vi "Register gRPC Messages.vi"(8 "error in (no error)":errorcluster, 11 "gRPC ID":T1) -> (0 "error out":errorcluster, 3 "gRPC ID Out":T1)   [LabVIEW 2025, in "xnet_can_bus_monitor_api_server.lvlib"]
uses:
  xnet_can_bus_monitor_api_server.lvlib
  <vilib>/gRPC/LabVIEW gRPC Library/Shared/grpcId.ctl
  <vilib>/gRPC/LabVIEW gRPC Library/Server API/typeDefs/Message Metadata.ctl
  <vilib>/gRPC/LabVIEW gRPC Library/Server API/typeDefs/Message Element Metadata.ctl
  <vilib>/gRPC/LabVIEW gRPC Library/Server API/typeDefs/Message Element Type.ctl
  <vilib>/gRPC/LabVIEW gRPC Library/Server API/typeDefs/Enum Metadata.ctl
  <vilib>/gRPC/LabVIEW gRPC Library/grpc-lvsupport-release.lvlib
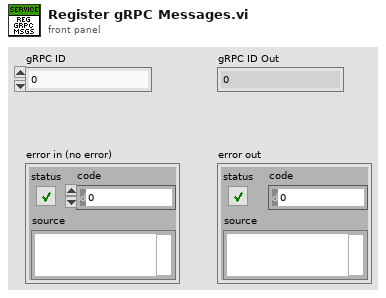
[diagram p1: front panel]
types:
  T1 = typedef "grpc-lvsupport-release.lvlib/grpcId.ctl" = u64
  T2 = typedef "grpc-lvsupport-release.lvlib/Enum Metadata.ctl" = cluster{"Version":i32, "Name":string, "Type Url":string, "Enum Values":string, "Allow Alias":bool}
  T3 = typedef "grpc-lvsupport-release.lvlib/Message Metadata.ctl" = cluster{"Version":i32, "Name":string, "Type Url":string, "Elements":T4[], "Has Oneof":bool}
  T4 = typedef "grpc-lvsupport-release.lvlib/Message Element Metadata.ctl" = cluster{"Field Name":string, "Embedded Message Name":string, "Protobuf Index":i32, "MessageElementType":T5, "Repeated":bool, "Is in Oneof":bool, "Oneof Container Name":string}
  T5 = typedef "grpc-lvsupport-release.lvlib/Message Element Type.ctl" = enum32{"Int32Value", "FloatValue", "DoubleValue", "BoolValue", "StringValue", "MessageValue", "Int64Value", "UInt32Value", "UInt64Value", "EnumValue", "Bytes", "Fixed64", "Fixed32", "SFixed64", "SFixed32", "SInt64", "SInt32"}
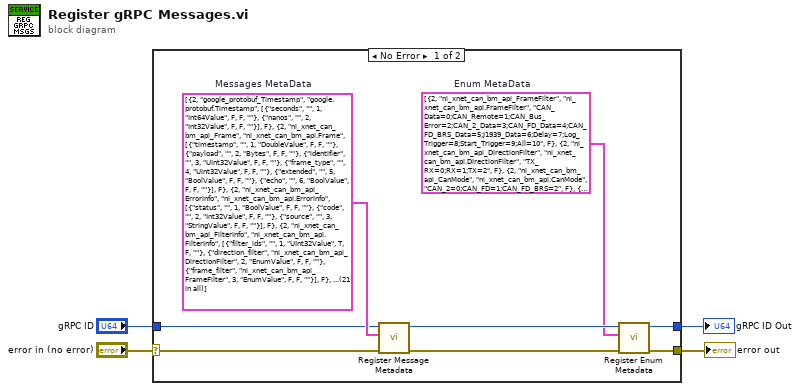
[diagram p0: block diagram]
diagram:
  n1 = case shown="No Error" "error in (no error)" {
    selector: "error in (no error)" -> [w10 w13]
    tunnel: [w9 w12] -> w2
    tunnel: [w6 w13] -> w1
    tunnel: "gRPC ID" -> [w9 w12]
    frame No Error {
      w5 = T2[] [{"Version"=2, "Name"="ni_xnet_can_bm_api_FrameFilter", "Type Url"="ni_xnet_can_bm_api.FrameFilter", "Enum Values"="CAN_Data=0;CAN_Remote=1;CAN_Bus_Error=2;CAN_2_Data=3;CAN_FD_Data=4;CAN_FD_BRS_Data=5;J1939_Data=6;Delay=7;Log_Trigger=8;Start_Trigger=9;All=10", "Allow Alias"=FALSE}, {"Version"=2, "Name"="ni_xnet_can_bm_api_DirectionFilter", "Type Url"="ni_xnet_can_bm_api.DirectionFilter", "Enum Values"="TX_RX=0;RX=1;TX=2", "Allow Alias"=FALSE}, {"Version"=2, "Name"="ni_xnet_can_bm_api_CanMode", "Type Url"="ni_xnet_can_bm_api.CanMode", "Enum Values"="CAN_2=0;CAN_FD=1;CAN_FD_BRS=2", "Allow Alias"=FALSE}, {"Version"=2, "Name"="ni_xnet_can_bm_api_CommState", "Type Url"="ni_xnet_can_bm_api.CommState", "Enum Values"="Error_Active=0;Error_Passive=1;Bus_Off=2;Init=3", "Allow Alias"=FALSE}, {"Version"=2, "Name"="ni_xnet_can_bm_api_LastCommError", "Type Url"="ni_xnet_can_bm_api.LastCommError", "Enum Values"="None=0;Stuff=1;Form=2;ACK=3;Bit1=4;Bit0=5;CRC=6", "Allow Alias"=FALSE}, {"Version"=2, "Name"="ni_xnet_can_bm_api_FdIsoMode", "Type Url"="ni_xnet_can_bm_api.FdIsoMode", "Enum Values"="ISO=0;Non_ISO=1;ISO_Legacy=2", "Allow Alias"=FALSE}, {"Version"=2, "Name"="ni_xnet_can_bm_api_Termination", "Type Url"="ni_xnet_can_bm_api.Termination", "Enum Values"="Term_Off=0;Term_On=1", "Allow Alias"=FALSE}]  # Enum MetaData
      w11 = T3[] [{"Version"=2, "Name"="google_protobuf_Timestamp", "Type Url"="google.protobuf.Timestamp", "Elements"=[{"Field Name"="seconds", "Embedded Message Name"="", "Protobuf Index"=1, "MessageElementType"=enum."Int64Value", "Repeated"=FALSE, "Is in Oneof"=FALSE, "Oneof Container Name"=""}, {"Field Name"="nanos", "Embedded Message Name"="", "Protobuf Index"=2, "MessageElementType"=enum."Int32Value", "Repeated"=FALSE, "Is in Oneof"=FALSE, "Oneof Container Name"=""}], "Has Oneof"=FALSE}, {"Version"=2, "Name"="ni_xnet_can_bm_api_Frame", "Type Url"="ni_xnet_can_bm_api.Frame", "Elements"=[{"Field Name"="timestamp", "Embedded Message Name"="", "Protobuf Index"=1, "MessageElementType"=enum."DoubleValue", "Repeated"=FALSE, "Is in Oneof"=FALSE, "Oneof Container Name"=""}, {"Field Name"="payload", "Embedded Message Name"="", "Protobuf Index"=2, "MessageElementType"=enum."Bytes", "Repeated"=FALSE, "Is in Oneof"=FALSE, "Oneof Container Name"=""}, {"Field Name"="identifier", "Embedded Message Name"="", "Protobuf Index"=3, "MessageElementType"=enum."UInt32Value", "Repeated"=FALSE, "Is in Oneof"=FALSE, "Oneof Container Name"=""}, {"Field Name"="frame_type", "Embedded Message Name"="", "Protobuf Index"=4, "MessageElementType"=enum."UInt32Value", "Repeated"=FALSE, "Is in Oneof"=FALSE, "Oneof Container Name"=""}, {"Field Name"="extended", "Embedded Message Name"="", "Protobuf Index"=5, "MessageElementType"=enum."BoolValue", "Repeated"=FALSE, "Is in Oneof"=FALSE, "Oneof Container Name"=""}, {"Field Name"="echo", "Embedded Message Name"="", "Protobuf Index"=6, "MessageElementType"=enum."BoolValue", "Repeated"=FALSE, "Is in Oneof"=FALSE, "Oneof Container Name"=""}], "Has Oneof"=FALSE}, {"Version"=2, "Name"="ni_xnet_can_bm_api_ErrorInfo", "Type Url"="ni_xnet_can_bm_api.ErrorInfo", "Elements"=[{"Field Name"="status", "Embedded Message Name"="", "Protobuf Index"=1, "MessageElementType"=enum."BoolValue", "Repeated"=FALSE, "Is in Oneof"=FALSE, "Oneof Container Name"=""}, {"Field Name"="code", "Embedded Message Name"="", "Protobuf Index"=2, "MessageElementType"=enum."Int32Value", "Repeated"=FALSE, "Is in Oneof"=FALSE, "Oneof Container Name"=""}, {"Field Name"="source", "Embedded Message Name"="", "Protobuf Index"=3, "MessageElementType"=enum."StringValue", "Repeated"=FALSE, "Is in Oneof"=FALSE, "Oneof Container Name"=""}], "Has Oneof"=FALSE}, {"Version"=2, "Name"="ni_xnet_can_bm_api_FilterInfo", "Type Url"="ni_xnet_can_bm_api.FilterInfo", "Elements"=[{"Field Name"="filter_ids", "Embedded Message Name"="", "Protobuf Index"=1, "MessageElementType"=enum."UInt32Value", "Repeated"=TRUE, "Is in Oneof"=FALSE, "Oneof Container Name"=""}, {"Field Name"="direction_filter", "Embedded Message Name"="ni_xnet_can_bm_api_DirectionFilter", "Protobuf Index"=2, "MessageElementType"=enum."EnumValue", "Repeated"=FALSE, "Is in Oneof"=FALSE, "Oneof Container Name"=""}, {"Field Name"="frame_filter", "Embedded Message Name"="ni_xnet_can_bm_api_FrameFilter", "Protobuf Index"=3, "MessageElementType"=enum."EnumValue", "Repeated"=FALSE, "Is in Oneof"=FALSE, "Oneof Container Name"=""}], "Has Oneof"=FALSE}, {"Version"=2, "Name"="ni_xnet_can_bm_api_ConnectSettings", "Type Url"="ni_xnet_can_bm_api.ConnectSettings", "Elements"=[{"Field Name"="port", "Embedded Message Name"="", "Protobuf Index"=1, "MessageElementType"=enum."StringValue", "Repeated"=FALSE, "Is in Oneof"=FALSE, "Oneof Container Name"=""}, {"Field Name"="can_mode", "Embedded Message Name"="ni_xnet_can_bm_api_CanMode", "Protobuf Index"=2, "MessageElementType"=enum."EnumValue", "Repeated"=FALSE, "Is in Oneof"=FALSE, "Oneof Container Name"=""}, {"Field Name"="termination", "Embedded Message Name"="ni_xnet_can_bm_api_Termination", "Protobuf Index"=3, "MessageElementType"=enum."EnumValue", "Repeated"=FALSE, "Is in Oneof"=FALSE, "Oneof Container Name"=""}, {"Field Name"="baud_rate", "Embedded Message Name"="", "Protobuf Index"=4, "MessageElementType"=enum."UInt64Value", "Repeated"=FALSE, "Is in Oneof"=FALSE, "Oneof Container Name"=""}, {"Field Name"="fd_baud_rate", "Embedded Message Name"="", "Protobuf Index"=5, "MessageElementType"=enum."UInt64Value", "Repeated"=FALSE, "Is in Oneof"=FALSE, "Oneof Container Name"=""}, {"Field Name"="fd_iso_mode", "Embedded Message Name"="ni_xnet_can_bm_api_FdIsoMode", "Protobuf Index"=6, "MessageElementType"=enum."EnumValue", "Repeated"=FALSE, "Is in Oneof"=FALSE, "Oneof Container Name"=""}], "Has Oneof"=FALSE}, {"Version"=2, "Name"="ni_xnet_can_bm_api_CanCommState", "Type Url"="ni_xnet_can_bm_api.CanCommState", "Elements"=[{"Field Name"="fault_code", "Embedded Message Name"="", "Protobuf Index"=1, "MessageElementType"=enum."Int32Value", "Repeated"=FALSE, "Is in Oneof"=FALSE, "Oneof Container Name"=""}, {"Field Name"="fault", "Embedded Message Name"="", "Protobuf Index"=2, "MessageElementType"=enum."BoolValue", "Repeated"=FALSE, "Is in Oneof"=FALSE, "Oneof Container Name"=""}, {"Field Name"="comm_state", "Embedded Message Name"="ni_xnet_can_bm_api_CommState", "Protobuf Index"=3, "MessageElementType"=enum."EnumValue", "Repeated"=FALSE, "Is in Oneof"=FALSE, "Oneof Container Name"=""}, {"Field Name"="last_comm_error", "Embedded Message Name"="ni_xnet_can_bm_api_LastCommError", "Protobuf Index"=4, "MessageElementType"=enum."EnumValue", "Repeated"=FALSE, "Is in Oneof"=FALSE, "Oneof Container Name"=""}, {"Field Name"="receive_error_counter", "Embedded Message Name"="", "Protobuf Index"=5, "MessageElementType"=enum."UInt32Value", "Repeated"=FALSE, "Is in Oneof"=FALSE, "Oneof Container Name"=""}, {"Field Name"="transmit_error_counter", "Embedded Message Name"="", "Protobuf Index"=6, "MessageElementType"=enum."UInt32Value", "Repeated"=FALSE, "Is in Oneof"=FALSE, "Oneof Container Name"=""}, {"Field Name"="transceiver_error", "Embedded Message Name"="", "Protobuf Index"=7, "MessageElementType"=enum."BoolValue", "Repeated"=FALSE, "Is in Oneof"=FALSE, "Oneof Container Name"=""}, {"Field Name"="sleep", "Embedded Message Name"="", "Protobuf Index"=8, "MessageElementType"=enum."BoolValue", "Repeated"=FALSE, "Is in Oneof"=FALSE, "Oneof Container Name"=""}], "Has Oneof"=FALSE}, {"Version"=2, "Name"="ni_xnet_can_bm_api_Session", "Type Url"="ni_xnet_can_bm_api.Session", "Elements"=[{"Field Name"="name", "Embedded Message Name"="", "Protobuf Index"=1, "MessageElementType"=enum."StringValue", "Repeated"=FALSE, "Is in Oneof"=FALSE, "Oneof Container Name"=""}, {"Field Name"="session_uid", "Embedded Message Name"="", "Protobuf Index"=2, "MessageElementType"=enum."StringValue", "Repeated"=FALSE, "Is in Oneof"=FALSE, "Oneof Container Name"=""}], "Has Oneof"=FALSE}, {"Version"=2, "Name"="ni_xnet_can_bm_api_PassThruRequest", "Type Url"="ni_xnet_can_bm_api.PassThruRequest", "Elements"=[{"Field Name"="session", "Embedded Message Name"="ni_xnet_can_bm_api_Session", "Protobuf Index"=1, "MessageElementType"=enum."MessageValue", "Repeated"=FALSE, "Is in Oneof"=FALSE, "Oneof Container Name"=""}, {"Field Name"="frame", "Embedded Message Name"="ni_xnet_can_bm_api_Frame", "Protobuf Index"=2, "MessageElementType"=enum."MessageValue", "Repeated"=FALSE, "Is in Oneof"=FALSE, "Oneof Container Name"=""}], "Has Oneof"=FALSE}, {"Version"=2, "Name"="ni_xnet_can_bm_api_PassThruReply", "Type Url"="ni_xnet_can_bm_api.PassThruReply", "Elements"=[{"Field Name"="error", "Embedded Message Name"="ni_xnet_can_bm_api_ErrorInfo", "Protobuf Index"=1, "MessageElementType"=enum."MessageValue", "Repeated"=FALSE, "Is in Oneof"=FALSE, "Oneof Container Name"=""}], "Has Oneof"=FALSE}, {"Version"=2, "Name"="ni_xnet_can_bm_api_GetStreamingFilterRequest", "Type Url"="ni_xnet_can_bm_api.GetStreamingFilterRequest", "Elements"=[{"Field Name"="session", "Embedded Message Name"="ni_xnet_can_bm_api_Session", "Protobuf Index"=1, "MessageElementType"=enum."MessageValue", "Repeated"=FALSE, "Is in Oneof"=FALSE, "Oneof Container Name"=""}], "Has Oneof"=FALSE}, {"Version"=2, "Name"="ni_xnet_can_bm_api_GetStreamingFilterReply", "Type Url"="ni_xnet_can_bm_api.GetStreamingFilterReply", "Elements"=[{"Field Name"="filter_info", "Embedded Message Name"="ni_xnet_can_bm_api_FilterInfo", "Protobuf Index"=1, "MessageElementType"=enum."MessageValue", "Repeated"=FALSE, "Is in Oneof"=FALSE, "Oneof Container Name"=""}, {"Field Name"="error", "Embedded Message Name"="ni_xnet_can_bm_api_ErrorInfo", "Protobuf Index"=2, "MessageElementType"=enum."MessageValue", "Repeated"=FALSE, "Is in Oneof"=FALSE, "Oneof Container Name"=""}], "Has Oneof"=FALSE}, {"Version"=2, "Name"="ni_xnet_can_bm_api_SetStreamingFilterRequest", "Type Url"="ni_xnet_can_bm_api.SetStreamingFilterRequest", "Elements"=[{"Field Name"="session", "Embedded Message Name"="ni_xnet_can_bm_api_Session", "Protobuf Index"=1, "MessageElementType"=enum."MessageValue", "Repeated"=FALSE, "Is in Oneof"=FALSE, "Oneof Container Name"=""}, {"Field Name"="filter_info", "Embedded Message Name"="ni_xnet_can_bm_api_FilterInfo", "Protobuf Index"=2, "MessageElementType"=enum."MessageValue", "Repeated"=FALSE, "Is in Oneof"=FALSE, "Oneof Container Name"=""}], "Has Oneof"=FALSE}, {"Version"=2, "Name"="ni_xnet_can_bm_api_SetStreamingFilterReply", "Type Url"="ni_xnet_can_bm_api.SetStreamingFilterReply", "Elements"=[{"Field Name"="error", "Embedded Message Name"="ni_xnet_can_bm_api_ErrorInfo", "Protobuf Index"=1, "MessageElementType"=enum."MessageValue", "Repeated"=FALSE, "Is in Oneof"=FALSE, "Oneof Container Name"=""}], "Has Oneof"=FALSE}, {"Version"=2, "Name"="ni_xnet_can_bm_api_ResetStreamingFilterRequest", "Type Url"="ni_xnet_can_bm_api.ResetStreamingFilterRequest", "Elements"=[{"Field Name"="session", "Embedded Message Name"="ni_xnet_can_bm_api_Session", "Protobuf Index"=1, "MessageElementType"=enum."MessageValue", "Repeated"=FALSE, "Is in Oneof"=FALSE, "Oneof Container Name"=""}], "Has Oneof"=FALSE}, {"Version"=2, "Name"="ni_xnet_can_bm_api_ResetStreamingFilterReply", "Type Url"="ni_xnet_can_bm_api.ResetStreamingFilterReply", "Elements"=[{"Field Name"="filter_info", "Embedded Message Name"="ni_xnet_can_bm_api_FilterInfo", "Protobuf Index"=1, "MessageElementType"=enum."MessageValue", "Repeated"=FALSE, "Is in Oneof"=FALSE, "Oneof Container Name"=""}, {"Field Name"="error", "Embedded Message Name"="ni_xnet_can_bm_api_ErrorInfo", "Protobuf Index"=2, "MessageElementType"=enum."MessageValue", "Repeated"=FALSE, "Is in Oneof"=FALSE, "Oneof Container Name"=""}], "Has Oneof"=FALSE}, {"Version"=2, "Name"="ni_xnet_can_bm_api_InitializeSettingsRequest", "Type Url"="ni_xnet_can_bm_api.InitializeSettingsRequest", "Elements"=[{"Field Name"="name", "Embedded Message Name"="", "Protobuf Index"=1, "MessageElementType"=enum."StringValue", "Repeated"=FALSE, "Is in Oneof"=FALSE, "Oneof Container Name"=""}, {"Field Name"="connect_settings", "Embedded Message Name"="ni_xnet_can_bm_api_ConnectSettings", "Protobuf Index"=2, "MessageElementType"=enum."MessageValue", "Repeated"=FALSE, "Is in Oneof"=FALSE, "Oneof Container Name"=""}, {"Field Name"="default_filter_ids", "Embedded Message Name"="", "Protobuf Index"=3, "MessageElementType"=enum."UInt32Value", "Repeated"=TRUE, "Is in Oneof"=FALSE, "Oneof Container Name"=""}], "Has Oneof"=FALSE}, {"Version"=2, "Name"="ni_xnet_can_bm_api_InitializeSettingsReply", "Type Url"="ni_xnet_can_bm_api.InitializeSettingsReply", "Elements"=[{"Field Name"="session", "Embedded Message Name"="ni_xnet_can_bm_api_Session", "Protobuf Index"=1, "MessageElementType"=enum."MessageValue", "Repeated"=FALSE, "Is in Oneof"=FALSE, "Oneof Container Name"=""}, {"Field Name"="error", "Embedded Message Name"="ni_xnet_can_bm_api_ErrorInfo", "Protobuf Index"=2, "MessageElementType"=enum."MessageValue", "Repeated"=FALSE, "Is in Oneof"=FALSE, "Oneof Container Name"=""}], "Has Oneof"=FALSE}, {"Version"=2, "Name"="ni_xnet_can_bm_api_StopProcessRequest", "Type Url"="ni_xnet_can_bm_api.StopProcessRequest", "Elements"=[{"Field Name"="session", "Embedded Message Name"="ni_xnet_can_bm_api_Session", "Protobuf Index"=1, "MessageElementType"=enum."MessageValue", "Repeated"=FALSE, "Is in Oneof"=FALSE, "Oneof Container Name"=""}], "Has Oneof"=FALSE}, {"Version"=2, "Name"="ni_xnet_can_bm_api_StopProcessReply", "Type Url"="ni_xnet_can_bm_api.StopProcessReply", "Elements"=[{"Field Name"="stopped", "Embedded Message Name"="", "Protobuf Index"=1, "MessageElementType"=enum."BoolValue", "Repeated"=FALSE, "Is in Oneof"=FALSE, "Oneof Container Name"=""}, {"Field Name"="error", "Embedded Message Name"="ni_xnet_can_bm_api_ErrorInfo", "Protobuf Index"=2, "MessageElementType"=enum."MessageValue", "Repeated"=FALSE, "Is in Oneof"=FALSE, "Oneof Container Name"=""}], "Has Oneof"=FALSE}, {"Version"=2, "Name"="ni_xnet_can_bm_api_StreamBusRequest", "Type Url"="ni_xnet_can_bm_api.StreamBusRequest", "Elements"=[{"Field Name"="session", "Embedded Message Name"="ni_xnet_can_bm_api_Session", "Protobuf Index"=1, "MessageElementType"=enum."MessageValue", "Repeated"=FALSE, "Is in Oneof"=FALSE, "Oneof Container Name"=""}], "Has Oneof"=FALSE}, {"Version"=2, "Name"="ni_xnet_can_bm_api_StreamBusReply", "Type Url"="ni_xnet_can_bm_api.StreamBusReply", "Elements"=[{"Field Name"="can_comm_state", "Embedded Message Name"="ni_xnet_can_bm_api_CanCommState", "Protobuf Index"=1, "MessageElementType"=enum."MessageValue", "Repeated"=FALSE, "Is in Oneof"=FALSE, "Oneof Container Name"=""}, {"Field Name"="frame", "Embedded Message Name"="ni_xnet_can_bm_api_Frame", "Protobuf Index"=2, "MessageElementType"=enum."MessageValue", "Repeated"=TRUE, "Is in Oneof"=FALSE, "Oneof Container Name"=""}, {"Field Name"="error", "Embedded Message Name"="ni_xnet_can_bm_api_ErrorInfo", "Protobuf Index"=3, "MessageElementType"=enum."MessageValue", "Repeated"=FALSE, "Is in Oneof"=FALSE, "Oneof Container Name"=""}], "Has Oneof"=FALSE}]  # Messages MetaData
      n2 = call <vilib>:"Register Message Metadata.vi"("error in"=w10, "Messages"=w11, "gRPCid in"=w9) -> ("error out"=w7:errorcluster, "gRPCid out"=w8:T1)  [unwired: 7 in]
      n3 = call <vilib>:"Register Enum Metadata.vi"("error in"=w7, "Enum Metadata"=w5, "gRPCid in"=w8) -> ("error out"=w6:errorcluster)  [unwired: 7 in, 1 out]
    }
    frame Error {
    }
  }
  "error out" <- w1
  "gRPC ID Out" <- w2
